vi "IncrementTime.vi"(0 "Factor":dbl, 1 "Position":cluster{"Card":dbl, "Channel":dbl}, 3 "Timing Array":refnum<vi>) -> ()   [LabVIEW 2013]
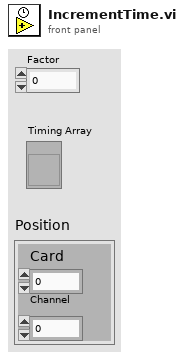
[diagram p1: front panel]
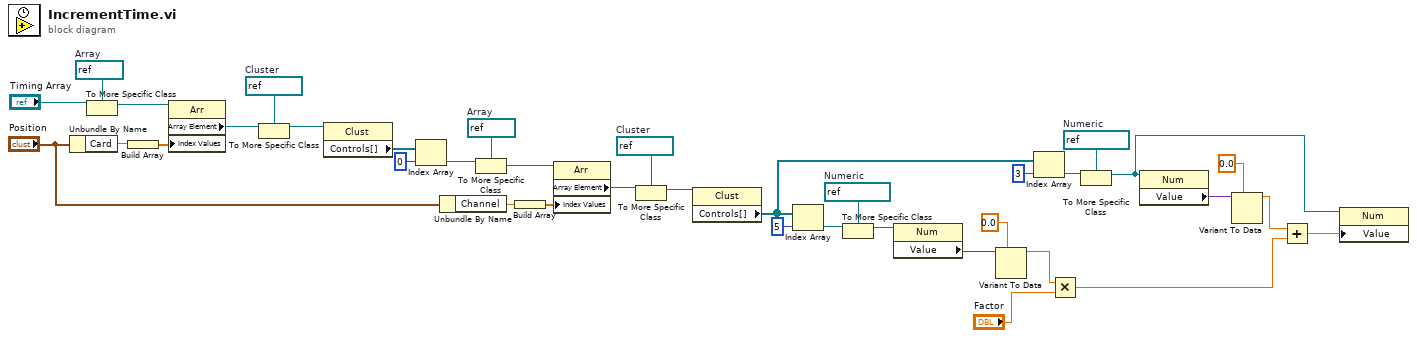
[diagram p0: block diagram]
diagram:
  w7 = refnum<vi> refnum  # Numeric
  w15 = refnum<vi> refnum  # Numeric
  w20 = refnum<vi> refnum  # Cluster
  w26 = refnum<vi> refnum  # Array
  w31 = refnum<vi> refnum  # Cluster
  w36 = refnum<vi> refnum  # Array
  n1 = Unbundle By Name("Position") -> ("Card"=w34:dbl)
  n2 = To More Specific Class(target class=w36, reference="Timing Array") -> (specific class reference=w35:refnum<vi>)  [unwired: 1 in, 1 out]
  n3 = Build Array(w34) -> (w33:dbl[])
  n4 = property class="Arr"(reference=w35, "Index Values"=w33) -> ("Array Element"=w32:refnum<vi>)  [unwired: 1 in, 2 out]
  n5 = To More Specific Class(target class=w31, reference=w32) -> (specific class reference=w30:refnum<vi>)  [unwired: 1 in, 1 out]
  n6 = property class="Clust"(reference=w30) -> ("Controls[]"=w29:refnum<vi>[])  [unwired: 1 in, 2 out]
  n7 = Index Array(array=w29, index=0) -> (element=w27:refnum<vi>)
  n8 = Unbundle By Name("Position") -> ("Channel"=w23:dbl)
  n9 = To More Specific Class(target class=w26, reference=w27) -> (specific class reference=w24:refnum<vi>)  [unwired: 1 in, 1 out]
  n10 = Build Array(w23) -> (w22:dbl[])
  n11 = property class="Arr"(reference=w24, "Index Values"=w22) -> ("Array Element"=w21:refnum<vi>)  [unwired: 1 in, 2 out]
  n12 = To More Specific Class(target class=w20, reference=w21) -> (specific class reference=w19:refnum<vi>)  [unwired: 1 in, 1 out]
  n13 = property class="Clust"(reference=w19) -> ("Controls[]"=w10:refnum<vi>[])  [unwired: 1 in, 2 out]
  n14 = Index Array(array=w10, index=5) -> (element=w16:refnum<vi>)
  n15 = To More Specific Class(target class=w15, reference=w16) -> (specific class reference=w14:refnum<vi>)  [unwired: 1 in, 1 out]
  n16 = property class="Num"(reference=w14) -> ("Value"=w13:variant)  [unwired: 1 in, 2 out]
  n17 = Variant To Data(type=0.0, Variant=w13) -> (data=w11:dbl)  [unwired: 1 in, 1 out]
  n18 = Index Array(array=w10, index=3) -> (element=w8:refnum<vi>)
  n19 = Multiply(x=w11, y="Factor") -> (x*y=w3:dbl)
  n20 = To More Specific Class(target class=w7, reference=w8) -> (specific class reference=w1:refnum<vi>)  [unwired: 1 in, 1 out]
  n21 = property class="Num"(reference=w1) -> ("Value"=w5:variant)  [unwired: 1 in, 2 out]
  n22 = Variant To Data(type=0.0, Variant=w5) -> (data=w4:dbl)  [unwired: 1 in, 1 out]
  n23 = Add(x=w4, y=w3) -> (x+y=w2:dbl)
  n24 = property class="Num"(reference=w1, "Value"=w2) -> ()  [unwired: 1 in, 2 out]
